vi "SeCrTs-DO Frequency  FGV.vi"(8 "error in":errorcluster, 9 "DO Set Frequency (W)":T1={"Samples to Read"=2000, "Pattern Mode?"=FALSE, "dt(sec)"=2000.0, "DO Init Time (Samples)"=2000, "dt per Read/Write"=2000.0, "Write Pointer"=2000, "Pattern Size"=2000, "Loop Rate (mSec)"=2000, "Buffer Size (Samples)"=2000, "Sampling rate"=2000.0, "Max DO Delay Time (samples)"=2000.0, "Min DO Delay Time (samples)"=2000.0, "Queue Size"=2000, "DO Init Sample Duration (Sec)"=2000.0}, 11 "Write/Read":T2=enum."Read") -> (0 "error in 2":errorcluster, 1 "DO Set Frequency (R)":T1={"Samples to Read"=2000, "Pattern Mode?"=FALSE, "dt(sec)"=2000.0, "DO Init Time (Samples)"=2000, "dt per Read/Write"=2000.0, "Write Pointer"=2000, "Pattern Size"=2000, "Loop Rate (mSec)"=2000, "Buffer Size (Samples)"=2000, "Sampling rate"=2000.0, "Max DO Delay Time (samples)"=2000.0, "Min DO Delay Time (samples)"=2000.0, "Queue Size"=2000, "DO Init Sample Duration (Sec)"=2000.0})   [LabVIEW 2022 SP3]
uses:
  RT Controls/ATF Storage-FGV Read write.ctl
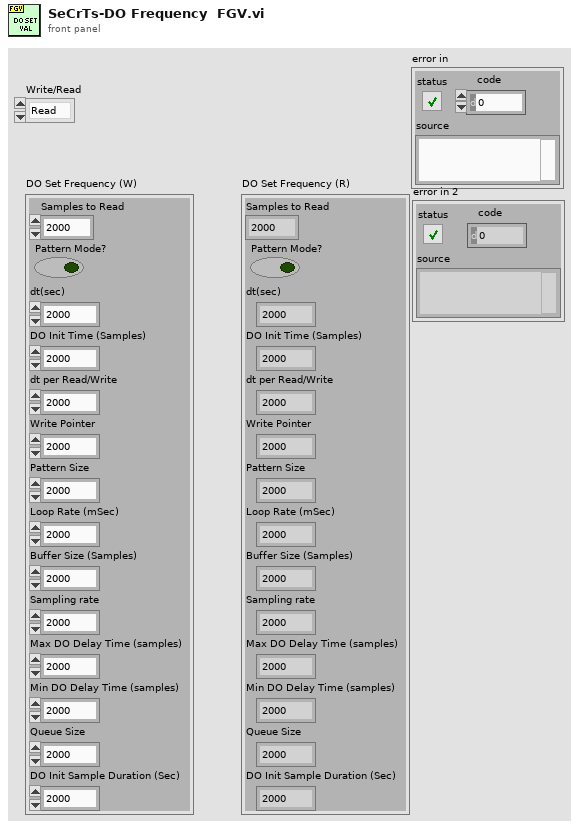
[diagram p1: front panel]
types:
  T1 = cluster{"Samples to Read":i32, "Pattern Mode?":bool, "dt(sec)":dbl, "DO Init Time (Samples)":i32, "dt per Read/Write":dbl, "Write Pointer":i32, "Pattern Size":i32, "Loop Rate (mSec)":i32, "Buffer Size (Samples)":i32, "Sampling rate":dbl, "Max DO Delay Time (samples)":dbl, "Min DO Delay Time (samples)":dbl, "Queue Size":i32, "DO Init Sample Duration (Sec)":dbl}
  T2 = typedef "ATF Storage-FGV Read write.ctl" = enum16{"Write", "Read"}
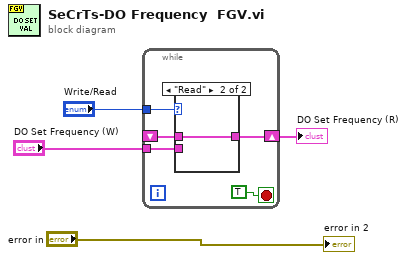
[diagram p0: block diagram]
diagram:
  n1 = while {
    tunnel: "Write/Read" -> [w8]
    shift-right: [w7] -> w2
    shift-left: _ -> [w6]
    tunnel: "DO Set Frequency (W)" -> [w5]
    stop <- TRUE stop-if-true
    n2 = case shown="\"Read\"" w8 {
      tunnel: [w10 w11] -> w7
      tunnel: w6 -> [_ w11]
      tunnel: w5 -> [w10 _]
      frame "Write" {
      }
      frame "Read" {
      }
    }
  }
  "DO Set Frequency (R)" <- w2
  "error in 2" <- "error in"
